vi "Cam-color3.vi"(7 "error in":errorcluster) -> (20 "Classifier Session (Color Classification 1)":T2, 21 "Classes (Color Classification 1)":string[](array[string]), 27 "error out":errorcluster)   [LabVIEW 2018]
uses:
  <vilib>/vision/Classification.llb/IMAQ Classifier Session.ctl
  <vilib>/userdefined/High Color/IMAQdx.ctl
  <vilib>/vision/Classification.llb/IMAQ Classifier Read Options.ctl
  <vilib>/vision/NI_Vision_Development_Module.lvlib
  <vilib>/vision/driver/NI_Vision_Acquisition_Software.lvlib
panel:
  in  "error in 2":errorcluster
  out "Image Out":T1(plugin-control)
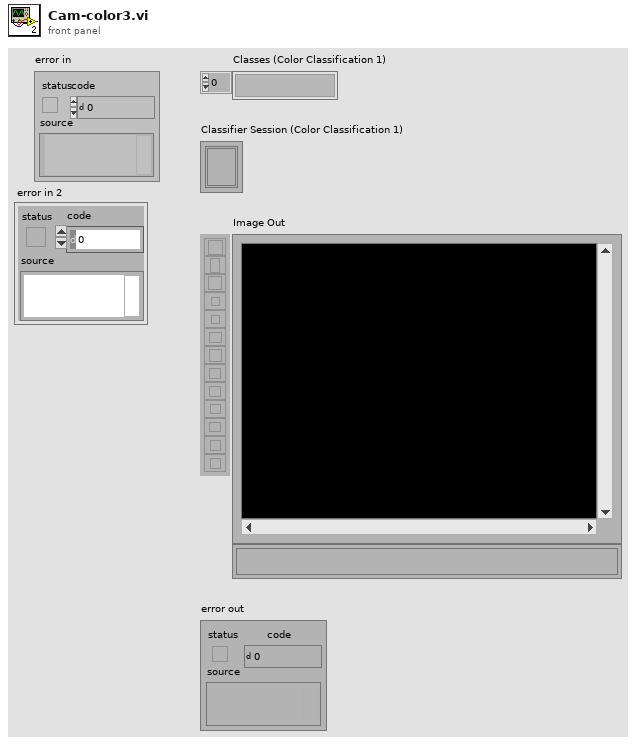
[diagram p1: front panel]
types:
  T1 = typedef "IMAQ Image.ctl" = refnum<image>
  T2 = typedef "IMAQ Classifier Session.ctl" = refnum<k1>
  T3 = typedef "IMAQdx.ctl" = refnum<k21>
  T4 = cluster{"Global Rectangle":i32[], "Contours":cluster{"ID":enum32{"External", "Internal"}, "Type":u32, "Coordinates":i32[]}[]}
  T5 = typedef "IMAQ Classifier Read Options.ctl" = i32
  T6 = typedef "ROI Descriptor" = cluster{"Global Rectangle":i32[], "Contours":cluster{"ID":enum32{"External", "Internal"}, "Type":u32, "Coordinates":i32[]}[]}
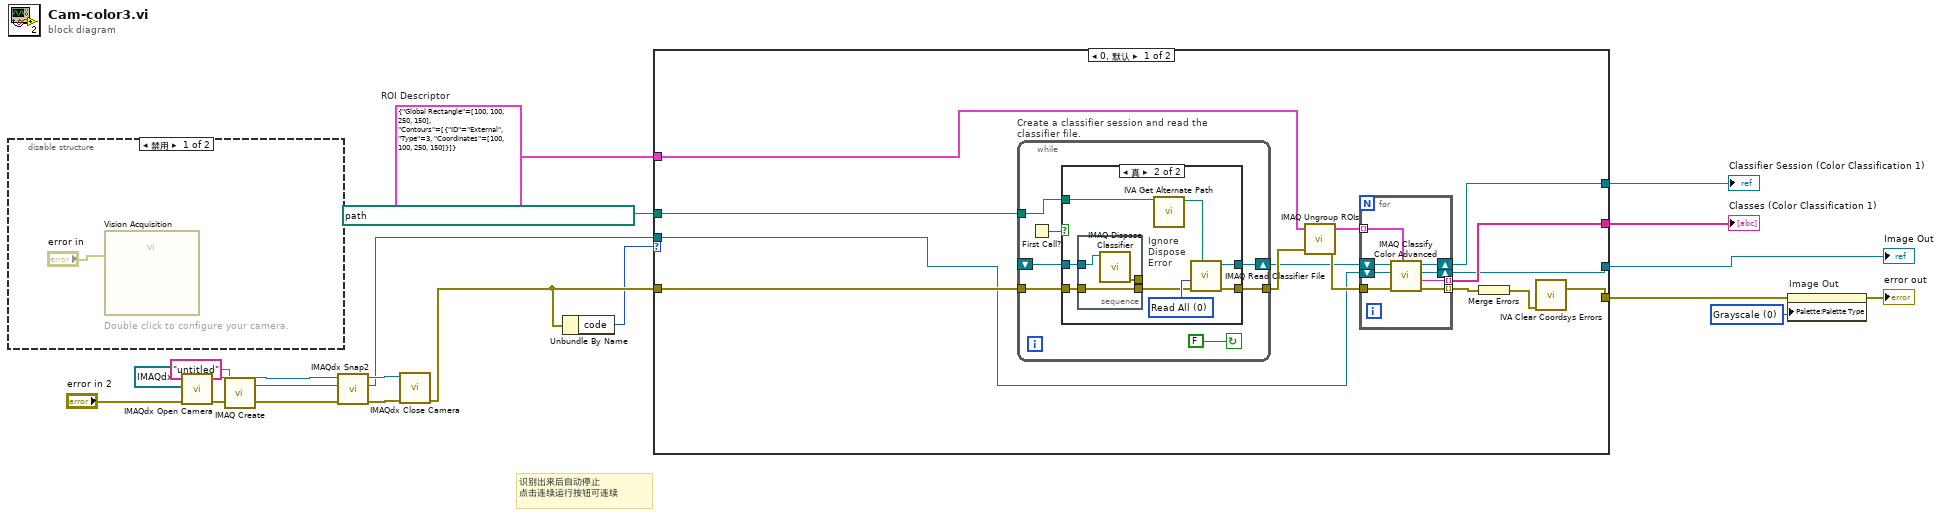
[diagram p0: block diagram]
diagram:
  w14 = u32 0 items=["Grayscale", "Binary", "Gradient", "Rainbow", "Temperature", "User Defined", "Binary 16 Bit", "Gradient 16 Bit", "Rainbow 16 Bit", "Temperature 16 Bit", "User Defined 16 Bit"] ("Palette Type")
  w19 = T4 {"Global Rectangle"=[100, 100, 250, 150], "Contours"=[{"ID"=enum."External", "Type"=3, "Coordinates"=[100, 100, 250, 150]}]}  # ROI Descriptor
  # "识别出来后自动停止\n点击连续运行按钮可连续"
  n1 = disable-structure shown="禁用" {
    frame Disabled {
      # "Double click to configure your camera."
      n2 = call "Vision Acquisition"("error in"="error in") -> ()  [unwired: 25 in, 2 out]
    }
    frame Enabled {
    }
  }
  n3 = call <vilib>:"IMAQdx Open Camera.vi"("error in"="error in 2", "Session In"=T3 "cam1") -> ("error out"=w13:errorcluster, "Session Out"=w10:T3)  [unwired: 8 in]
  n4 = call "IMAQ Create"("Image Name"="untitled", "error in (no error)"=w13) -> ("New Image"=w8:T1, "error out"=w12:errorcluster)  [unwired: 3 in]
  n5 = call <vilib>:"IMAQdx Snap2.vi"("error in"=w12, "Image In"=w8, "Session In"=w10) -> ("error out"=w11:errorcluster, "Image Out"=w5:T1, "Session Out"=w9:T3)  [unwired: 6 in]
  n6 = call <vilib>:"IMAQdx Close Camera.vi"("error in"=w11, "Session In"=w9) -> ("error out"=w2:errorcluster)  [unwired: 9 in]
  n7 = Unbundle By Name(w2) -> ("code"=w1:i32)
  n8 = case shown="0, 默认" w1 {
    tunnel: [w35 _] -> w20
    tunnel: w19 -> [w34 _]
    tunnel: [w28 _] -> w18
    tunnel: [w26 _] -> w17
    tunnel: [w25 _] -> w15
    tunnel: w2 -> [w24 _]
    tunnel: w5 -> [w23 _]
    tunnel: path "D:/Labviewprogram/视觉/视觉框架/Color 识别.clf" ("File Path") -> [w22 _]
    frame 0, Default {
      n9 = while "Create a classifier session and read the classifier file." {
        shift-right: [w50] -> w27
        shift-left: _ -> [w49]
        tunnel: w24 -> [w47]
        tunnel: [w46] -> w33
        tunnel: w22 -> [w44]
        stop <- FALSE continue-if-true
        n10 = First Call?() -> (First Call?: T/F=w45:bool)
        n11 = case "条件结构" shown="真" w45 {
          tunnel: [w52 w59] -> w50
          tunnel: w49 -> [w52 w57]
          tunnel: w47 -> [w51 w56]
          tunnel: [w51 w58] -> w46
          tunnel: w44 -> [_ w54]
          frame False {
          }
          frame True {
            w60 = T5 0 items=["Read All", "Add Samples, Do Not Change Options", "Read Options, Do Not Add Samples"] ("Read Options")
            # "Ignore Dispose Error"
            n12 = stacked-sequence "层叠式顺序结构" {
              tunnel: w57 -> [w63]
              tunnel: w56 -> [w62]
              tunnel: [w62] -> w55
              tunnel: [w61] -> _
              frame #0 {
                n13 = call "IMAQ Dispose Classifier"("Classifier Session"=w63) -> ("error out"=w61:errorcluster)  [unwired: 1 in, 9 out]
              }
            }
            n14 = call <vilib>:"IVA Get Alternate Path.vi"("Path In"=w54) -> ("Path Out"=w53:path)  [unwired: 10 out]
            n15 = call "IMAQ Read Classifier File"("File Path"=w53, "error in (no error)"=w55, "Read Options"=w60) -> ("error out"=w58:errorcluster, "Classifier Session"=w59:T2)  [unwired: 1 in, 6 out]
          }
        }
      }
      n16 = call "IMAQ Ungroup ROIs"("error in (no error)"=w33, "ROI Descriptor"=w34) -> ("error out"=w32:errorcluster, "ROI Descriptors out"=w31:T6[])  [unwired: 2 out]
      n17 = for "For循环" {
        tunnel: [w43] -> w35 mode=indexing
        tunnel: [w42] -> w30 mode=indexing
        tunnel: w32 -> [w40]
        tunnel: w31 -> [w39] mode=indexing
        shift-right: [w37] -> w25
        shift-left: w23 -> [w38]
        shift-right: [w36] -> w26
        shift-left: w27 -> [w41]
        n18 = call "IMAQ Classify Color Advanced"("ROI Descriptor"=w39, "error in (no error)"=w40, "Image"=w38, "Classifier Session"=w41) -> ("error out"=w42:errorcluster, "Class"=w43:string, "Image (dup)"=w37:T1, "Classifier Session (dup)"=w36:T2)  [unwired: 4 out]
      }
      n19 = Merge Errors(w30) -> (w29:errorcluster)
      n20 = call <vilib>:"IVA Clear Coordsys Errors.vi"("error in (no error)"=w29) -> ("error out"=w28:errorcluster)  [unwired: 10 in]
    }
    frame 1 {
    }
  }
  "Classes (Color Classification 1)" <- w20
  "Classifier Session (Color Classification 1)" <- w17
  "Image Out" <- w15
  n21 = property on="Image Out" class="ImageControl"(error in=w18, "Palette:Palette Type"=w14) -> (error out=→"error out":errorcluster)  [unwired: 1 in, 1 out]
